vi "Initialize.vi"(7 "not in use":string="Setpoint.ch%d.SP", 8 "error in":errorcluster, 9 "Number of Channels":u32=1, 10 "Instance Name":string, 11 "Cycler in":refnum<class "Cycler.lvclass">) -> (0 "error out":errorcluster, 3 "Cycler out":refnum<class "Cycler.lvclass">)   [LabVIEW 2023, in "Cycler.lvclass"]
uses:
  Cycler.lvclass
  Cycler.lvclass/Cycler.ctl
  Low Level Capabilities/OnOff/OnOff.lvclass
  Low Level Capabilities/Output Enable/Output Enable.lvclass
  Low Level Capabilities/Control Mode/Control Mode.lvclass
  Low Level Capabilities/Current/Current Actual Value/Current Actual Value.lvclass
  Low Level Capabilities/Current/Current Gradient/Current Gradient.lvclass
  Low Level Capabilities/Current/Current Limit/Current Limit.lvclass
  Low Level Capabilities/Current/Current Setpoint/Current Setpoint.lvclass
  Low Level Capabilities/Power/Power Actual Value/Power Actual Value.lvclass
  Low Level Capabilities/Power/Power Gradient/Power Gradient.lvclass
  Low Level Capabilities/Power/Power Limit/Power Limit.lvclass
  Low Level Capabilities/Power/Power Setpoint/Power Setpoint.lvclass
  Low Level Capabilities/Voltage/Voltage Actual Value/Voltage Actual Value.lvclass
  Low Level Capabilities/Voltage/Voltage Gradient/Voltage Gradient.lvclass
  Low Level Capabilities/Voltage/Voltage Limit/Voltage Limit.lvclass
  Low Level Capabilities/Voltage/Voltage Setpoint/Voltage Setpoint.lvclass
  Low Level Capabilities/Error/Error.lvclass
  Low Level Capabilities/Error Channels/Error Channels.lvclass
  Low Level Capabilities/Iso Measurement/Iso Measurement.lvclass
  Low Level Capabilities/Parallel Mode/Parallel Mode.lvclass
  Low Level Capabilities/Parameter Set/Parameter Set.lvclass
  Low Level Capabilities/Current/Current Nominal Value/Current Nominal Value.lvclass
  Low Level Capabilities/Power/Power Nominal Value/Power Nominal Value.lvclass
  Low Level Capabilities/Voltage/Voltage Nominal Value/Voltage Nominal Value.lvclass
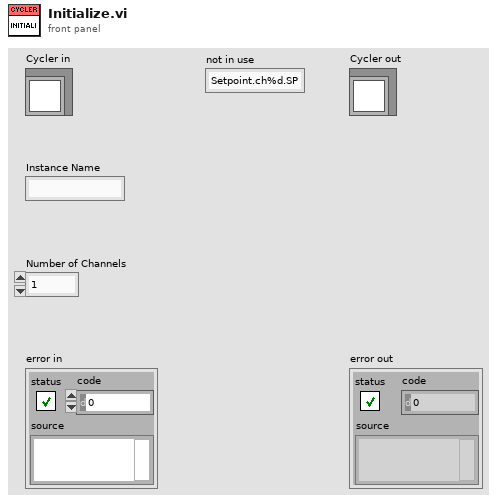
[diagram p1: front panel]
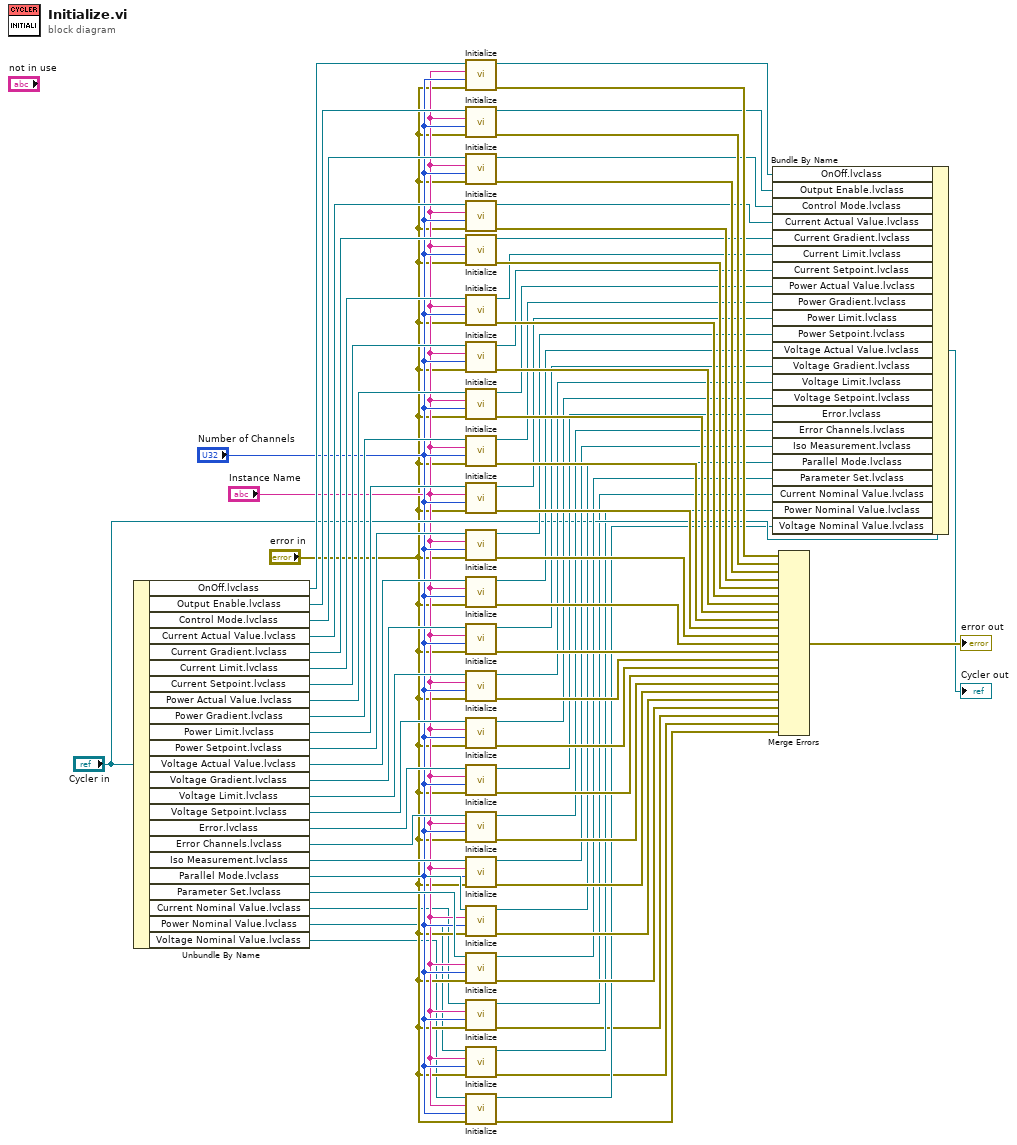
[diagram p0: block diagram]
diagram:
  n1 = Unbundle By Name("Cycler in") -> ("OnOff.lvclass"=w75:refnum<class "OnOff.lvclass">, "Output Enable.lvclass"=w72:refnum<class "Output Enable.lvclass">, "Control Mode.lvclass"=w69:refnum<class "Control Mode.lvclass">, "Current Actual Value.lvclass"=w66:refnum<class "Current Actual Value.lvclass">, "Current Gradient.lvclass"=w63:refnum<class "Current Gradient.lvclass">, "Current Limit.lvclass"=w60:refnum<class "Current Limit.lvclass">, "Current Setpoint.lvclass"=w57:refnum<class "Current Setpoint.lvclass">, "Power Actual Value.lvclass"=w54:refnum<class "Power Actual Value.lvclass">, "Power Gradient.lvclass"=w51:refnum<class "Power Gradient.lvclass">, "Power Limit.lvclass"=w48:refnum<class "Power Limit.lvclass">, "Power Setpoint.lvclass"=w45:refnum<class "Power Setpoint.lvclass">, "Voltage Actual Value.lvclass"=w42:refnum<class "Voltage Actual Value.lvclass">, "Voltage Gradient.lvclass"=w39:refnum<class "Voltage Gradient.lvclass">, "Voltage Limit.lvclass"=w36:refnum<class "Voltage Limit.lvclass">, "Voltage Setpoint.lvclass"=w33:refnum<class "Voltage Setpoint.lvclass">, "Error.lvclass"=w30:refnum<class "Error.lvclass">, "Error Channels.lvclass"=w27:refnum<class "Error Channels.lvclass">, "Iso Measurement.lvclass"=w24:refnum<class "Iso Measurement.lvclass">, "Parallel Mode.lvclass"=w19:refnum<class "Parallel Mode.lvclass">, "Parameter Set.lvclass"=w18:refnum<class "Parameter Set.lvclass">, "Current Nominal Value.lvclass"=w9:refnum<class "Current Nominal Value.lvclass">, "Power Nominal Value.lvclass"=w8:refnum<class "Power Nominal Value.lvclass">, "Voltage Nominal Value.lvclass"=w7:refnum<class "Voltage Nominal Value.lvclass">)
  n2 = call-dynamic "Initialize.vi"("error in"="error in", "Number of Channels"="Number of Channels", "Instance Name"="Instance Name", "OnOff in"=w75) -> ("error out"=w73:errorcluster, "OnOff out"=w74:refnum<class "OnOff.lvclass">)  [unwired: 6 in]
  n3 = call-dynamic "Initialize.vi"("error in"="error in", "Number of Channels"="Number of Channels", "Instance Name"="Instance Name", "Output Enable in"=w72) -> ("error out"=w70:errorcluster, "Output Enable out"=w71:refnum<class "Output Enable.lvclass">)  [unwired: 6 in]
  n4 = call-dynamic "Initialize.vi"("error in"="error in", "Number of Channels"="Number of Channels", "Instance Name"="Instance Name", "Control Mode in"=w69) -> ("error out"=w68:errorcluster, "Control Mode out"=w67:refnum<class "Control Mode.lvclass">)  [unwired: 6 in]
  n5 = call-dynamic "Initialize.vi"("error in"="error in", "Number of Channels"="Number of Channels", "Instance Name"="Instance Name", "Current Actual Value in"=w66) -> ("error out"=w65:errorcluster, "Current Actual Value out"=w64:refnum<class "Current Actual Value.lvclass">)  [unwired: 6 in]
  n6 = call-dynamic "Initialize.vi"("error in"="error in", "Number of Channels"="Number of Channels", "Instance Name"="Instance Name", "Current Gradient in"=w63) -> ("error out"=w62:errorcluster, "Current Gradient out"=w61:refnum<class "Current Gradient.lvclass">)  [unwired: 6 in]
  n7 = call-dynamic "Initialize.vi"("error in"="error in", "Number of Channels"="Number of Channels", "Instance Name"="Instance Name", "Current Limit in"=w60) -> ("error out"=w58:errorcluster, "Current Limit out"=w59:refnum<class "Current Limit.lvclass">)  [unwired: 6 in]
  n8 = call-dynamic "Initialize.vi"("error in"="error in", "Number of Channels"="Number of Channels", "Instance Name"="Instance Name", "Current Setpoint in"=w57) -> ("error out"=w56:errorcluster, "Current Setpoint out"=w55:refnum<class "Current Setpoint.lvclass">)  [unwired: 6 in]
  n9 = call-dynamic "Initialize.vi"("error in"="error in", "Number of Channels"="Number of Channels", "Instance Name"="Instance Name", "Power Actual Value in"=w54) -> ("error out"=w53:errorcluster, "Power Actual Value out"=w52:refnum<class "Power Actual Value.lvclass">)  [unwired: 6 in]
  n10 = call-dynamic "Initialize.vi"("error in"="error in", "Number of Channels"="Number of Channels", "Instance Name"="Instance Name", "Power Gradient in"=w51) -> ("error out"=w49:errorcluster, "Power Gradient out"=w50:refnum<class "Power Gradient.lvclass">)  [unwired: 6 in]
  n11 = call-dynamic "Initialize.vi"("error in"="error in", "Number of Channels"="Number of Channels", "Instance Name"="Instance Name", "Power Limit in"=w48) -> ("error out"=w47:errorcluster, "Power Limit out"=w46:refnum<class "Power Limit.lvclass">)  [unwired: 6 in]
  n12 = call-dynamic "Initialize.vi"("error in"="error in", "Number of Channels"="Number of Channels", "Instance Name"="Instance Name", "Power Setpoint in"=w45) -> ("error out"=w44:errorcluster, "Power Setpoint out"=w43:refnum<class "Power Setpoint.lvclass">)  [unwired: 6 in]
  n13 = call-dynamic "Initialize.vi"("error in"="error in", "Number of Channels"="Number of Channels", "Instance Name"="Instance Name", "Voltage Actual Value in"=w42) -> ("error out"=w40:errorcluster, "Voltage Actual Value out"=w41:refnum<class "Voltage Actual Value.lvclass">)  [unwired: 6 in]
  n14 = call-dynamic "Initialize.vi"("error in"="error in", "Number of Channels"="Number of Channels", "Instance Name"="Instance Name", "Voltage Gradient in"=w39) -> ("error out"=w37:errorcluster, "Voltage Gradient out"=w38:refnum<class "Voltage Gradient.lvclass">)  [unwired: 6 in]
  n15 = call-dynamic "Initialize.vi"("error in"="error in", "Number of Channels"="Number of Channels", "Instance Name"="Instance Name", "Voltage Limit in"=w36) -> ("error out"=w35:errorcluster, "Voltage Limit out"=w34:refnum<class "Voltage Limit.lvclass">)  [unwired: 6 in]
  n16 = call-dynamic "Initialize.vi"("error in"="error in", "Number of Channels"="Number of Channels", "Instance Name"="Instance Name", "Voltage Setpoint in"=w33) -> ("error out"=w31:errorcluster, "Voltage Setpoint out"=w32:refnum<class "Voltage Setpoint.lvclass">)  [unwired: 6 in]
  n17 = call-dynamic "Initialize.vi"("error in"="error in", "Number of Channels"="Number of Channels", "Instance Name"="Instance Name", "Error in"=w30) -> ("error out"=w28:errorcluster, "Error out"=w29:refnum<class "Error.lvclass">)  [unwired: 6 in]
  n18 = call-dynamic "Initialize.vi"("error in"="error in", "Number of Channels"="Number of Channels", "Instance Name"="Instance Name", "Error Channels in"=w27) -> ("error out"=w26:errorcluster, "Error Channels out"=w25:refnum<class "Error Channels.lvclass">)  [unwired: 6 in]
  n19 = call-dynamic "Initialize.vi"("error in"="error in", "Number of Channels"="Number of Channels", "Instance Name"="Instance Name", "Iso Measurement in"=w24) -> ("error out"=w22:errorcluster, "Iso Measurement out"=w23:refnum<class "Iso Measurement.lvclass">)  [unwired: 6 in]
  n20 = call-dynamic "Initialize.vi"("error in"="error in", "Number of Channels"="Number of Channels", "Instance Name"="Instance Name", "Parallel Mode in"=w19) -> ("error out"=w21:errorcluster, "Parallel Mode out"=w20:refnum<class "Parallel Mode.lvclass">)  [unwired: 6 in]
  n21 = call-dynamic "Initialize.vi"("error in"="error in", "Number of Channels"="Number of Channels", "Instance Name"="Instance Name", "Parameter Set in"=w18) -> ("error out"=w16:errorcluster, "Parameter Set out"=w17:refnum<class "Parameter Set.lvclass">)  [unwired: 6 in]
  n22 = call-dynamic "Initialize.vi"("error in"="error in", "Number of Channels"="Number of Channels", "Instance Name"="Instance Name", "Current Nominal Value in"=w9) -> ("error out"=w3:errorcluster, "Current Nominal Value out"=w6:refnum<class "Current Nominal Value.lvclass">)  [unwired: 6 in]
  n23 = call-dynamic "Initialize.vi"("error in"="error in", "Number of Channels"="Number of Channels", "Instance Name"="Instance Name", "Power Nominal Value in"=w8) -> ("error out"=w2:errorcluster, "Power Nominal Value out"=w5:refnum<class "Power Nominal Value.lvclass">)  [unwired: 6 in]
  n24 = call-dynamic "Initialize.vi"("error in"="error in", "Number of Channels"="Number of Channels", "Instance Name"="Instance Name", "Voltage Nominal Value in"=w7) -> ("error out"=w1:errorcluster, "Voltage Nominal Value out"=w4:refnum<class "Voltage Nominal Value.lvclass">)  [unwired: 6 in]
  n25 = Bundle By Name(cluster="Cycler in", "OnOff.lvclass"=w74, "Output Enable.lvclass"=w71, "Control Mode.lvclass"=w67, "Current Actual Value.lvclass"=w64, "Current Gradient.lvclass"=w61, "Current Limit.lvclass"=w59, "Current Setpoint.lvclass"=w55, "Power Actual Value.lvclass"=w52, "Power Gradient.lvclass"=w50, "Power Limit.lvclass"=w46, "Power Setpoint.lvclass"=w43, "Voltage Actual Value.lvclass"=w41, "Voltage Gradient.lvclass"=w38, "Voltage Limit.lvclass"=w34, "Voltage Setpoint.lvclass"=w32, "Error.lvclass"=w29, "Error Channels.lvclass"=w25, "Iso Measurement.lvclass"=w23, "Parallel Mode.lvclass"=w20, "Parameter Set.lvclass"=w17, "Current Nominal Value.lvclass"=w6, "Power Nominal Value.lvclass"=w5, "Voltage Nominal Value.lvclass"=w4) -> (→"Cycler out":refnum<class "Cycler.lvclass">)
  n26 = Merge Errors(w73, w70, w68, w65, w62, w58, w56, w53, w49, w47, w44, w40, w37, w35, w31, w28, w26, w22, w21, w16, w3, w2, w1) -> (→"error out":errorcluster)
